vi "saveLogEntry.vi"(8 "error in (no error)":errorcluster, 11 "Logger in":refnum<class "Log.lvclass">) -> (0 "error out":errorcluster, 3 "Logger out":refnum<class "Log.lvclass">)   [LabVIEW 2013, in "Log.lvclass"]
uses:
  Log.lvclass
  Log.lvclass/Log.ctl
  <vilib>/Utility/file.llb/Write To Spreadsheet File (string).vi
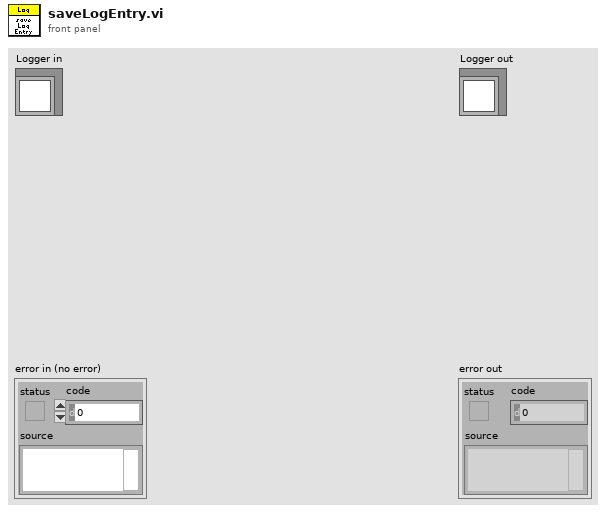
[diagram p1: front panel]
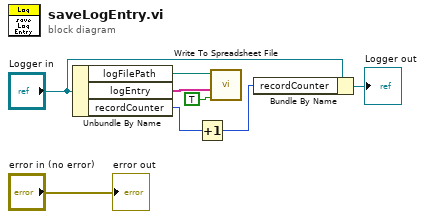
[diagram p0: block diagram]
diagram:
  n1 = Unbundle By Name("Logger in") -> ("logFilePath"=w7:path, "logEntry"=w1:string[], "recordCounter"=w6:u32)
  n2 = Increment(x=w6) -> (x+1=w5:u32)
  n3 = call-poly <vilib>:"Write To Spreadsheet File.vi"("append to file? (new file:F)"=TRUE, "1D data"=w1, "file path (dialog if empty)"=w7) -> ()  [unwired: 5 in, 1 out]
  n4 = Bundle By Name(cluster="Logger in", "recordCounter"=w5) -> (→"Logger out":refnum<class "Log.lvclass">)
  "error out" <- "error in (no error)"
